vi "Memory write from DMA - Host.vi"(8 "error in":errorcluster, 11 "FPGA VI Reference In":refnum<k20>) -> (0 "error out":errorcluster, 3 "FPGA VI Reference Out":refnum<k20>, 4 "Write memory complete":bool, 6 "FXP Init Data Out":fxp<+/-,12,12>[](array[numeric]))   [LabVIEW 2014]
uses:
  <vilib>/rvi/interface/common/niFpgaWaitOnOcc.vi
  <vilib>/Utility/error.llb/Error Cluster From Error Code.vi
  <vilib>/rvi/errors/niLvFpgaAdjustHostInterfaceError.vi
  <vilib>/RVI Host/nirviSupport.llb/nirviErrorClusterFromErrorCode.vi
  <vilib>/rvi/interface/nirviMethod/nirviMethod.xnode
  <vilib>/FPGAPlugInAG/Dynamic/niLvFpga_WriteFifo_Dynamic.vi
  <vilib>/rvi/errors/niLvFpgaMergeErrorWithErrorCode.vi
  <vilib>/FPGAPlugInAG/Dynamic/niLvFpga_StartFifo_Dynamic.vi
  <vilib>/FPGAPlugInAG/Dynamic/niLvFpga_ConfigureFifo_Dynamic.vi
  <vilib>/rvi/interface/nirviMethod/StockFPGA_InlinedMethodWaitForSingleIRQ.vi
  <vilib>/FPGAPlugInAG/Dynamic/niLvFpga_WaitOnIrq_Dynamic.vi
  <vilib>/FPGAPlugInAG/Dynamic/niLvFpga_AcknowledgeIrq_Dynamic.vi
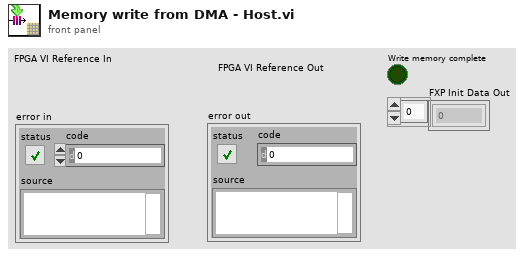
[diagram p1: front panel]
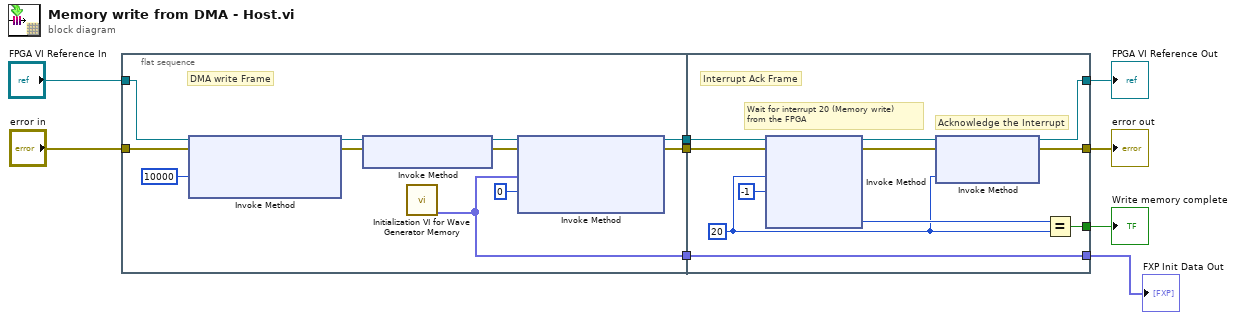
[diagram p0: block diagram]
diagram:
  n1 = flat-sequence {
    tunnel: [w14] -> w9
    tunnel: [w13] -> w6
    tunnel: "error in" -> [w12]
    tunnel: "FPGA VI Reference In" -> [w11]
    tunnel: [w10] -> w2
    tunnel: [w25] -> w7
    tunnel: [w26] -> w8
    tunnel: w9 -> [w30]
    tunnel: w6 -> [w31]
    tunnel: [w22] -> w5
    tunnel: [w21] -> w1
    tunnel: w2 -> [w21]
    frame #0 {
      # "DMA write Frame"
      n2 = xnode "Invoke Method"("FPGA VI Reference In"=w11, "error in"=w12, "Requested Depth"=u32 10000) -> ("FPGA VI Reference Out"=w19:refnum<k20>, "error out"=w18:errorcluster)  [unwired: 1 out]
      n3 = xnode "Invoke Method"("FPGA VI Reference In"=w19, "error in"=w18) -> ("FPGA VI Reference Out"=w16:refnum<k20>, "error out"=w17:errorcluster)
      n4 = call "Initialization VI for Wave Generator Memory.vi"() -> ("FXP Init Data Out"=w10:fxp<+/-,12,12>[])  [unwired: 10 in, 1 out]
      n5 = xnode "Invoke Method"("FPGA VI Reference In"=w16, "error in"=w17, "Data"=w10, "Timeout (ms)"=0) -> ("FPGA VI Reference Out"=w14:refnum<k20>, "error out"=w13:errorcluster)  [unwired: 1 out]
    }
    frame #1 {
      w23 = 20 ("IRQ Number(s)")
      # "Acknowledge the Interrupt"
      # "Wait for interrupt 20 (Memory write)\nfrom the FPGA"
      # "Interrupt Ack Frame"
      n6 = xnode "Invoke Method"("FPGA VI Reference In"=w30, "error in"=w31, "IRQ Number(s)"=w23, "Timeout (ms)"=-1) -> ("FPGA VI Reference Out"=w27:refnum<k20>, "error out"=w28:errorcluster, "IRQ(s) Asserted"=w24:i32)  [unwired: 1 out]
      n7 = xnode "Invoke Method"("FPGA VI Reference In"=w27, "error in"=w28, "IRQ Number(s)"=w23) -> ("FPGA VI Reference Out"=w25:refnum<k20>, "error out"=w26:errorcluster)
      n8 = Equal?(x=w24, y=w23) -> (x = y?=w22:bool)
    }
  }
  "error out" <- w8
  "FPGA VI Reference Out" <- w7
  "Write memory complete" <- w5
  "FXP Init Data Out" <- w1
